vi "CSM Module Template - Tiny.vi"(7 "Name (\"\" to Use UUID)":string="CSM Tiny") -> ()   [LabVIEW 2017]
doc: "Compact code template for creating a CSM module without a user interface. The functionality of this template is identical to the CSM Module Template VI.\n\n\n> [!NOTE] <b>CSM Naming Rules</b>\n>\n> - CSM module name must be unique. Otherwise, CSM enters a `Critical Error` state.\n> - If the input module name is an empty string (\"\"), the system uses a UUID as the module name. Such a module is marked as standalone mode and does not appear in the module list.\n> - Worker Mode Rule: If the input module name ends with `#`, a worker mode node will be instantiated. Multiple worker mode nodes can form a worker mode module.\n> - Chain of Responsibility Mode Rule: If the input module name ends with `$` followed by a number, a chain of responsibility mode node will be instantiated. Multiple chain of responsibility mode nodes can form a chain of responsibility mode module.\n> - System-Level Module Rule: If the input module name starts with `.`, the module is a system-level module. Under default settings, such modules are not listed by the CSM - List Modules VI and are suitable for instantiating modules that run in the background.\n> - Submodule Rule: `.` is also allowed in a module name to separate the module name into multiple parts. CSM does not have strict rules for submodules. The `.` in the module name only marks the logical relationship between different modules. From an execution perspective, they are considered independent modules. The only difference is that you can obtain a list of logical submodules via the CSM - List Submodules VI.\n\n\n-- <b>Controls</b> --\n- <b>Name (\"\" to use UUID)</b>: CSM module name. Refer to <b>CSM Naming Rules</b> for module naming rules."
uses:
  user.lib/_NEVSTOP/Communicable State Machine(CSM)/AdvanceAPI/CSM - Revert Arguments-Safe String.vi
  user.lib/_NEVSTOP/Communicable State Machine(CSM)/AdvanceAPI/CSM - Break Down Multiple States String.vi
  user.lib/_NEVSTOP/Communicable State Machine(CSM)/AdvanceAPI/CSM - Compact Multiple States.vi
  user.lib/_NEVSTOP/Communicable State Machine(CSM)/AdvanceAPI/CSM - Make String Arguments Safe.vi
  user.lib/_NEVSTOP/Communicable State Machine(CSM)/AdvanceAPI/CSM - Keywords.vi
  user.lib/_NEVSTOP/Communicable State Machine(CSM)/_Shared/Trim Single-line Text.vi
  user.lib/_NEVSTOP/Communicable State Machine(CSM)/Communicable State Machine.lvlib
panel:
  in  "Exit":bool
  out "State History":string
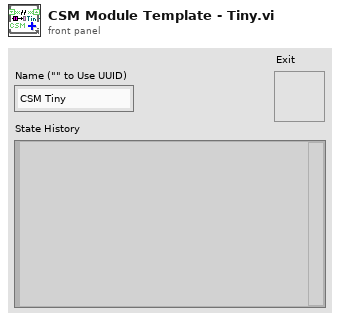
[diagram p1: front panel]
types:
  T1 = enum32{"Invalid", "Standard", "Closed", "Hidden", "Minimized", "Maximized"}
  T2 = enum32{"invalid app kind", "Development System", "Run Time System", "Student Edition", "Embedded LabVIEW", "Evaluation", "Custom"}
  T3 = typedef "Communicable State Machine.lvlib/_CSM_Response Source Message.ctl" = cluster{"‘State":string, "’Arguments":string, "’Error":errorcluster}
  T4 = cluster{"Current VI Reference":refnum<vi>, "Close Panel on Exit?":bool}
  T5 = cluster{"Core":cluster{"Current VI Reference":refnum<vi>, "Close Panel on Exit?":bool}, "Your Boolean data":bool, "Your string data":string}
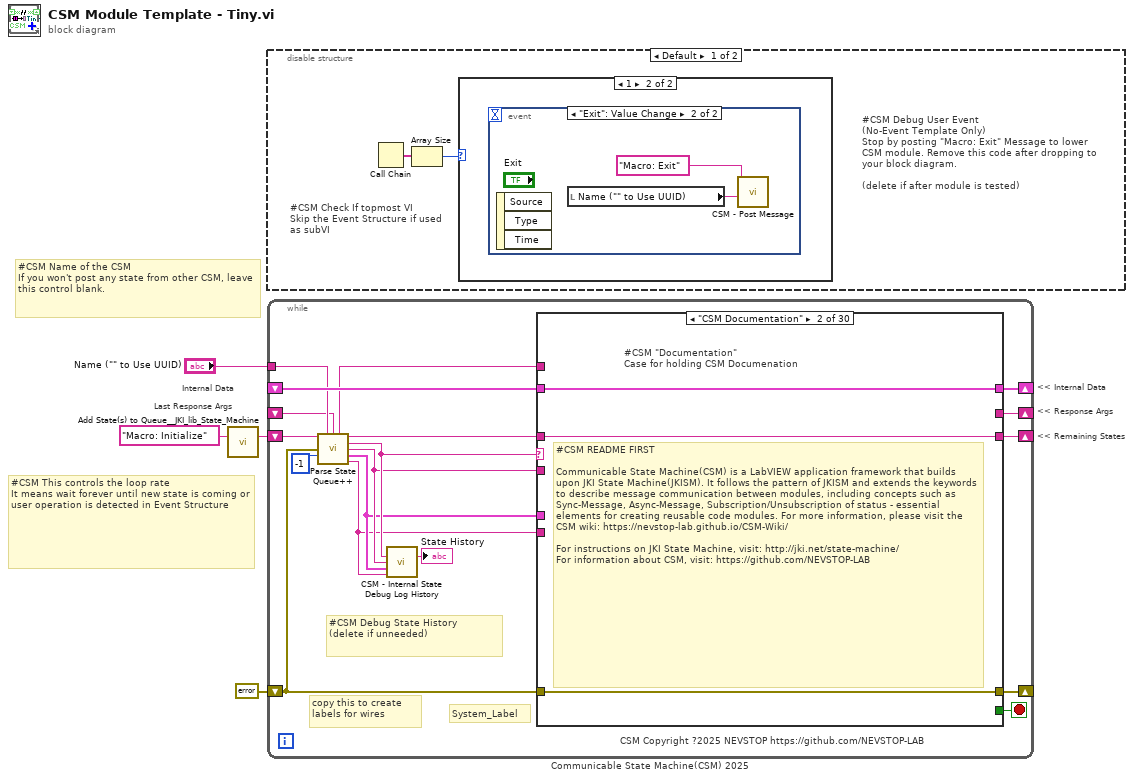
[diagram p0: block diagram]
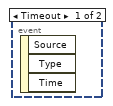
[diagram p3: hidden frame]
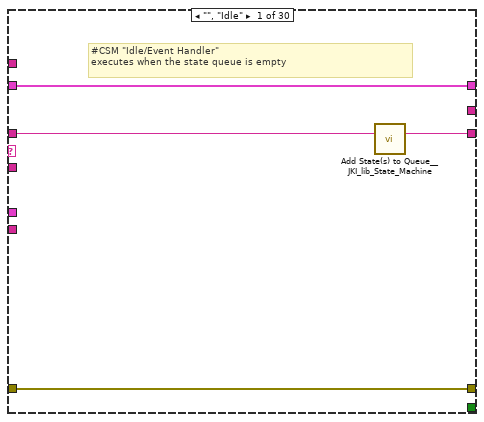
[diagram p5: hidden frame]
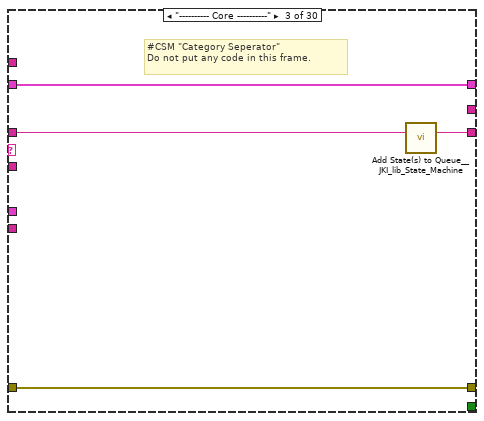
[diagram p6: hidden frame]
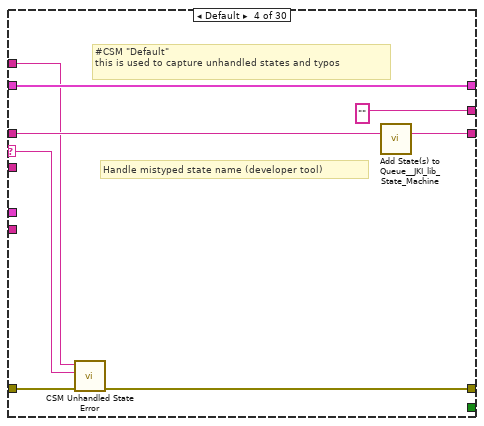
[diagram p7: hidden frame]
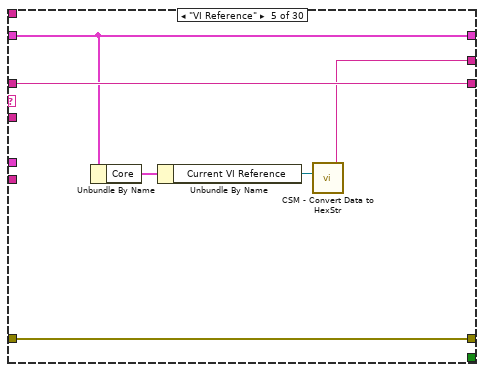
[diagram p8: hidden frame]
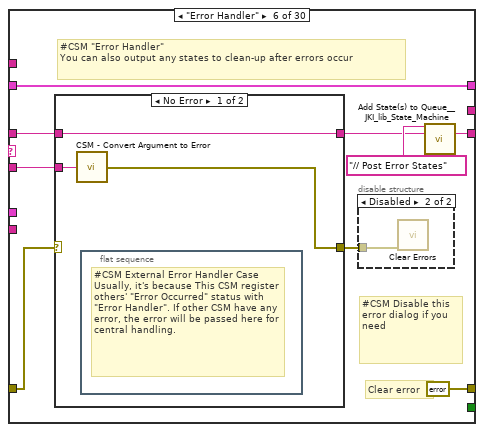
[diagram p9: hidden frame]
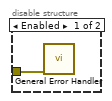
[diagram p10: hidden frame]
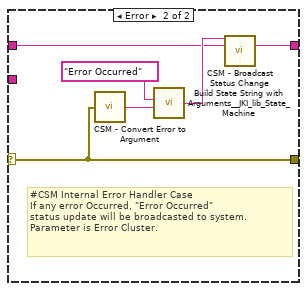
[diagram p11: hidden frame]
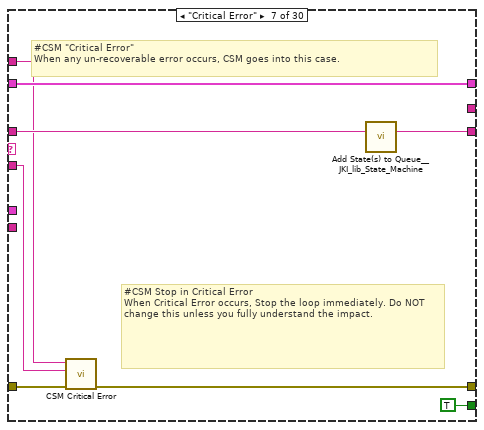
[diagram p12: hidden frame]
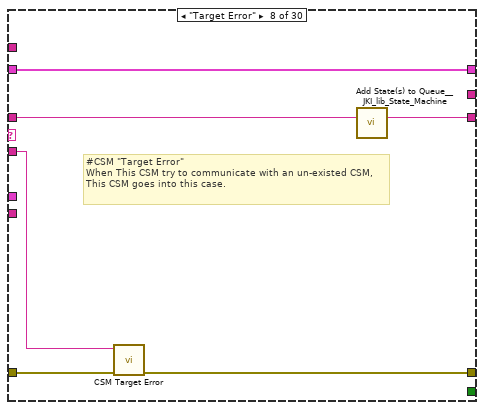
[diagram p13: hidden frame]
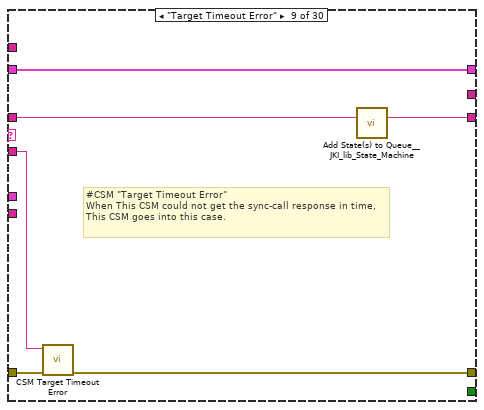
[diagram p14: hidden frame]
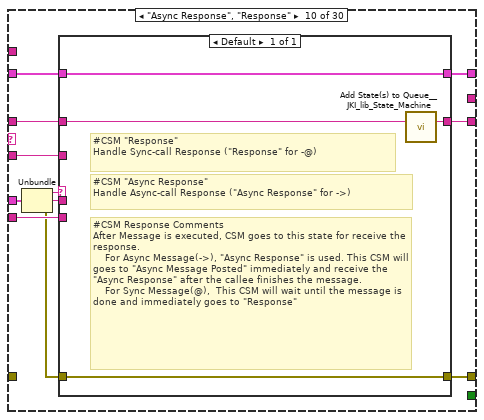
[diagram p15: hidden frame]
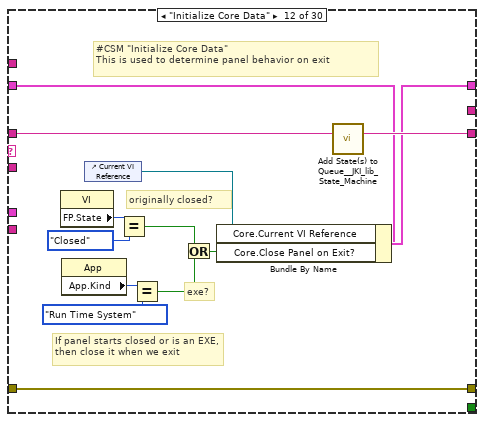
[diagram p17: hidden frame]
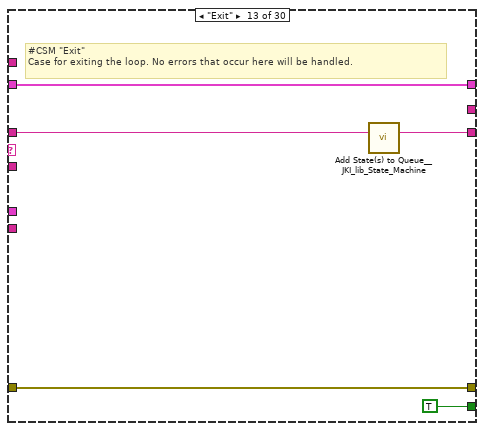
[diagram p18: hidden frame]
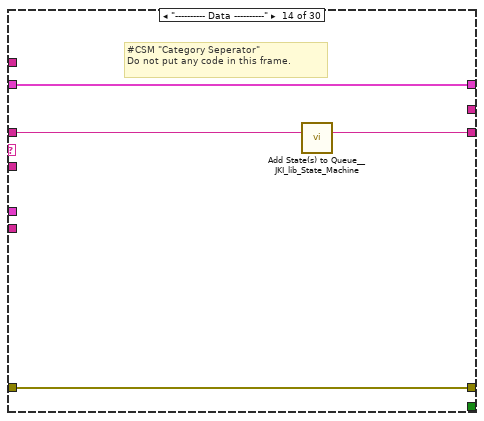
[diagram p19: hidden frame]
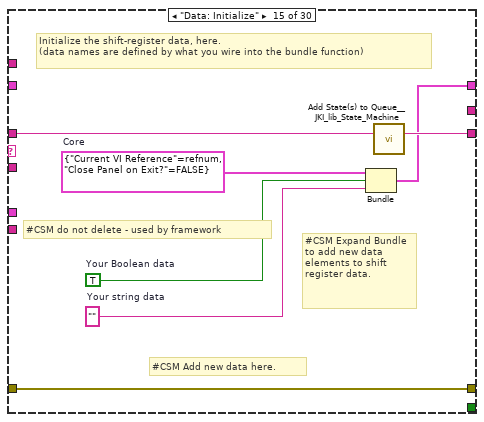
[diagram p20: hidden frame]
diagram:
  # "Last Response Args"
  # "Internal Data"
  # "#CSM Name of the CSM\nIf you won't post any state from other CSM, leave this control blank."
  # "#CSM This controls the loop rate\nIt means wait forever until new state is coming or user operation is detected in Event Structure"
  # "<< Internal Data"
  # "<< Response Args"
  # "<< Remaining States"
  n1 = call <vilib>:"Add State(s) to Queue__JKI_lib_State_Machine.vi"("State(s) in (\"\")"="Macro: Initialize" ("Init State(\"Macro: Initialize\")")) -> ("States Out"=w4:string)  [unwired: 14 in]
  n2 = disable-structure shown="Default" {
    frame condition #0 (active) {
      # "#CSM Check If topmost VI\nSkip the Event Structure if used as subVI"
      # "#CSM Debug User Event\n(No-Event Template Only)\nStop by posting \"Macro: Exit\" Message to lower CSM module. Remove this code after dropping to your block diagram. \n\n(delete if after module is tested)"
      n3 = Call Chain() -> (call chain=w6:string[])
      n4 = Array Size(array=w6) -> (size(s)=w5:i32)
      n5 = case shown="1" w5 {
        frame Default {
        }
        frame 1 {
          n6 = event shown="[1] \"Exit\": Value Change" {
            selector: _ -> [_ _]
            dyn-events: _ -> [_ _]
            timeout: _ -> [_ _]
            event Timeout {
              n7 = event-data() -> ()  [unwired: 1 in, 3 out]
            }
            event "Exit": Value Change {
              n8 = event-data() -> ()  [unwired: 1 in, 3 out]
              n9 = local read "Name (\"\" to Use UUID)"() -> (w8:string)
              n10 = call "CSM - Post Message.vi"("Target Module"=w8, "State"="Macro: Exit" ("States")) -> ()  [unwired: 9 in, 1 out]
            }
          }
        }
      }
    }
    frame condition #1 {
    }
  }
  n11 = while "Communicable State Machine(CSM) 2025" {
    shift-right: [w21] -> _
    shift-left: _ -> [w20]
    shift-right: [w24] -> _
    shift-left: errorcluster {"status"=FALSE, "code"=0, "source"=""} ("error out") -> [w19]
    shift-right: [w23] -> _
    shift-left: w4 -> [w25]
    tunnel: "Name (\"\" to Use UUID)" -> [w17]
    shift-right: [w18] -> _
    shift-left: _ -> [w11]
    stop <- w22 stop-if-true
    # "#CSM Debug State History\n(delete if unneeded)"
    # "copy this to create labels for wires"
    # "System_Label"
    # "CSM Copyright ?2025 NEVSTOP https://github.com/NEVSTOP-LAB"
    n12 = call "Parse State Queue++.vi"("State Queue"=w25, "Name (\"\" to Use UUID)"=w17, "Response Arguments"=w11, "Previous Error"=w19, "Dequeue (1 ms)"=-1 ("Timeout")) -> ("Name Used"=w12:string, "Remaining States"=w26:string, "Current State"=w16:string, "Arguments"=w15:string, "Additional Information"=w14:T3, "Source CSM"=w13:string)  [unwired: 5 in]
    n13 = call "CSM - Internal State Debug Log History.vi"("State"=w16, "Arguments (\"\")"=w15, ">> Response Source Message >>"=w14, "Source (\"\")"=w13) -> ("Debug Log"=→"State History":string)  [unwired: 11 in]
    n14 = case shown="\"CSM Documentation\"" w16 {
      selector: w16 -> [_ _ _ w40 _ _ _ _ _ _ _ _ _ _ _ _ _ _ _ _ _ _ _ _ _ _ _ _ _ _]
      tunnel: w26 -> [w27 w32 w37 w44 w50 w56 w77 w83 w89 w97 w108 w122 w127 w131 w138 w140 w147 w151 w155 w161 w176 w245 w250 w257 w259 w263 w268 w275 w279 w283]
      tunnel: w15 -> [_ _ _ _ _ w55 w73 w82 w87 w96 _ _ _ _ _ _ _ _ _ w156 w170 _ _ _ _ _ w266 _ _ _]
      tunnel: w20 -> [w28 w31 w34 w42 w49 w59 w78 w84 w90 w99 w107 w115 w125 w128 _ w139 w142 w148 w153 w159 w172 w242 w247 w254 w258 w262 w267 w272 w276 w280]
      tunnel: [w29 w33 w35 w38 w51 errorcluster {"status"=FALSE, "code"=0, "source"=""} ("error out") w74 w80 w86 w102 w109 w119 w124 w129 w135 w141 w143 w149 w152 w157 w173 w243 w248 w255 w260 w264 w269 w273 w277 w281] -> w24
      tunnel: w19 -> [w29 w33 w35 w45 w51 w57 w79 w81 w88 _ w109 w119 w124 w129 w135 w141 w144 w149 w152 w158 w174 w243 w248 w255 w260 w264 w269 w273 w277 w281]
      tunnel: [w30 w32 w36 w43 w50 w52 w76 w85 w91 w98 w108 w121 w126 w130 w137 w140 w146 w150 w154 w160 w175 w244 w249 w256 w259 w263 w268 w274 w278 w282] -> w23
      tunnel: [_ _ _ _ _ _ TRUE _ _ _ _ _ TRUE _ _ _ _ _ _ _ _ _ _ _ _ _ _ _ _ _] -> w22
      tunnel: [w28 w31 w34 w42 w49 w59 w78 w84 w90 w100 w107 w120 w125 w128 w136 w139 w142 w148 w153 w159 w172 w242 w247 w254 w258 w262 w267 w272 w276 w280] -> w21
      tunnel: w13 -> [_ _ _ _ _ _ _ _ _ w94 _ _ _ _ _ _ _ _ _ _ _ _ _ _ _ _ _ _ _ _]
      tunnel: w14 -> [_ _ _ _ _ _ _ _ _ w101 _ _ _ _ _ _ _ _ _ _ _ _ _ _ _ _ _ _ _ _]
      tunnel: [_ _ _ "" w46 _ _ _ _ _ _ _ _ _ _ _ _ _ _ _ _ _ _ _ _ "API1 Response" w265 _ _ _] -> w18
      tunnel: w12 -> [_ _ _ w39 _ _ w72 _ _ _ _ _ _ _ _ _ _ _ _ _ _ _ _ _ _ _ _ _ _ _]
      frame "", "Idle" {
        # "#CSM \"Idle/Event Handler\"\nexecutes when the state queue is empty"
        n15 = call <vilib>:"Add State(s) to Queue__JKI_lib_State_Machine.vi"("State(s) in (\"\")"=w27) -> ("States Out"=w30:string)  [unwired: 14 in]
      }
      frame "CSM Documentation" {
        # "#CSM README FIRST\n\nCommunicable State Machine(CSM) is a LabVIEW application framework that builds upon JKI State Machine(JKISM). It follows the pattern of JKISM and extends the keywords to describe message communication between modules, including concepts such as Sync-Message, Async-Message, Subscription/Unsubscription of status - essential elements for creating reusable code modules. For more information, please visit the CSM wiki: https://nevstop-lab.github.io/CSM-Wiki/\n\nFor instructions on JKI State Machine, visit: http://jki.net/state-machine/\nFor information about CSM, visit: https://github.com/NEVSTOP-LAB"
        # "#CSM \"Documentation\"\nCase for holding CSM Documenation"
      }
      frame "---------- Core ----------" {
        # "#CSM \"Category Seperator\"\nDo not put any code in this frame."
        n16 = call <vilib>:"Add State(s) to Queue__JKI_lib_State_Machine.vi"("State(s) in (\"\")"=w37) -> ("States Out"=w36:string)  [unwired: 14 in]
      }
      frame Default {
        # "#CSM \"Default\"\nthis is used to capture unhandled states and typos"
        # "Handle mistyped state name (developer tool)"
        n17 = call "CSM Unhandled State Error.vi"("error in (no error)"=w45, "Undefined State"=w40, "CSM Name"=w39) -> ("error out"=w38:errorcluster)  [unwired: 8 in]
        n18 = call <vilib>:"Add State(s) to Queue__JKI_lib_State_Machine.vi"("State(s) in (\"\")"=w44) -> ("States Out"=w43:string)  [unwired: 14 in]
      }
      frame "VI Reference" {
        n19 = Unbundle By Name(w49) -> ("Core"=w48:T4)
        n20 = Unbundle By Name(w48) -> ("Current VI Reference"=w47:refnum<vi>)
        n21 = call "CSM - Convert Data to HexStr.vi"("Variant"=w47) -> ("HEX String (0-9,A-F)"=w46:string)  [unwired: 8 in]
      }
      frame "Error Handler" {
        # "#CSM Disable this error dialog if you need"
        # "#CSM \"Error Handler\"\nYou can also output any states to clean-up after errors occur"
        # "Clear error"
        n22 = case shown="No Error" w57 {
          selector: w57 -> [_ w66]
          tunnel: [w65 w68] -> w53
          tunnel: w56 -> [w65 w67]
          tunnel: w55 -> [w64 _]
          tunnel: [w63 w66] -> w58
          frame No Error {
            n23 = call "CSM - Convert Argument to Error.vi"("Argument"=w64) -> ("Error"=w63:errorcluster)  [unwired: 4 in]
            n24 = flat-sequence {
              frame #0 {
                # "#CSM External Error Handler Case\nUsually, it's because This CSM register others' \"Error Occurred\" status with \"Error Handler\". If other CSM have any error, the error will be passed here for central handling."
              }
            }
          }
          frame Error {
            # "#CSM Internal Error Handler Case \nIf any error Occurred, \"Error Occurred\" \nstatus update will be broadcasted to system.\nParameter is Error Cluster."
            n25 = call "CSM - Convert Error to Argument.vi"("Error"=w66) -> ("Argument"=w70:string)  [unwired: 4 in]
            n26 = call <vilib>:"Build State String with Arguments__JKI_lib_State_Machine.vi"("Arguments (\"\")"=w70, "State"="Error Occurred" ("Status with Arguments")) -> ("State with Arguments"=w69:string)  [unwired: 4 in]
            n27 = call "CSM - Broadcast Status Change.vi"("Status With Arguments"=w69, "State Queue"=w67) -> ("Remaining States"=w68:string)  [unwired: 13 in]
          }
        }
        n28 = disable-structure shown="Disabled" {
          disable-tunnel: w58 -> [w61 w62]
          frame Enabled {
            n29 = call <vilib>:"General Error Handler.vi"("error in (no error)"=w61) -> ()  [unwired: 10 in, 5 out]
          }
          frame Disabled {
            n30 = call <vilib>:"Clear Errors.vi"("error in (no error)"=w62) -> ()  [unwired: 5 in, 2 out]
          }
        }
        n31 = call <vilib>:"Add State(s) to Queue__JKI_lib_State_Machine.vi"("State(s) in Front (\"\")"="// Post Error States", "State(s) in (\"\")"=w53) -> ("States Out"=w52:string)  [unwired: 13 in]
      }
      frame "Critical Error" {
        # "#CSM Stop in Critical Error\nWhen Critical Error occurs, Stop the loop immediately. Do NOT change this unless you fully understand the impact."
        # "#CSM \"Critical Error\"\nWhen any un-recoverable error occurs, CSM goes into this case."
        n32 = call "CSM Critical Error.vi"("error in (no error)"=w79, "Arugments (As Reason)"=w73, "CSM Name"=w72) -> ("error out"=w74:errorcluster)  [unwired: 8 in]
        n33 = call <vilib>:"Add State(s) to Queue__JKI_lib_State_Machine.vi"("State(s) in (\"\")"=w77) -> ("States Out"=w76:string)  [unwired: 14 in]
      }
      frame "Target Error" {
        # "#CSM \"Target Error\"\nWhen This CSM try to communicate with an un-existed CSM, This CSM goes into this case."
        n34 = call "CSM Target Error.vi"("error in (no error)"=w81, "Arguments (As CSM Name)"=w82) -> ("error out"=w80:errorcluster)  [unwired: 9 in]
        n35 = call <vilib>:"Add State(s) to Queue__JKI_lib_State_Machine.vi"("State(s) in (\"\")"=w83) -> ("States Out"=w85:string)  [unwired: 14 in]
      }
      frame "Target Timeout Error" {
        # "#CSM \"Target Timeout Error\"\nWhen This CSM could not get the sync-call response in time, This CSM goes into this case."
        n36 = call "CSM Target Timeout Error.vi"("error in (no error)"=w88, "Arguments (As CSM Name)"=w87) -> ("error out"=w86:errorcluster)  [unwired: 9 in]
        n37 = call <vilib>:"Add State(s) to Queue__JKI_lib_State_Machine.vi"("State(s) in (\"\")"=w89) -> ("States Out"=w91:string)  [unwired: 14 in]
      }
      frame "Async Response", "Response" {
        n38 = Unbundle(w101) -> ("‘State"=w95:string, "’Arguments"=w93:string, "’Error"=w92:errorcluster)
        n39 = case shown="Default" w95 {
          tunnel: [w106] -> w102
          tunnel: w92 -> [w106]
          tunnel: [w105] -> w100
          tunnel: w99 -> [w105]
          tunnel: [w103] -> w98
          tunnel: w97 -> [w104]
          tunnel: w96 -> [_]
          tunnel: w94 -> [_]
          tunnel: w93 -> [_]
          frame Default {
            # "#CSM Response Comments\nAfter Message is executed, CSM goes to this state for receive the response.\n    For Async Message(->), \"Async Response\" is used. This CSM will goes to \"Async Message Posted\" immediately and receive the \"Async Response\" after the callee finishes the message.\n    For Sync Message(@),  This CSM will wait until the message is done and immediately goes to \"Response\""
            # "#CSM \"Async Response\"\nHandle Async-call Response (\"Async Response\" for ->)"
            # "#CSM \"Response\"\nHandle Sync-call Response (\"Response\" for -@)"
            n40 = call <vilib>:"Add State(s) to Queue__JKI_lib_State_Machine.vi"("State(s) in (\"\")"=w104) -> ("States Out"=w103:string)  [unwired: 14 in]
          }
        }
      }
      frame "Async Message Posted" {
        # "#CSM \"Async Message Posted\"\nAfter Async Message is posted (-> or ->| ), CSM goes to this state for post-action.\nYou can use Argument - State to tell which Async Message is called."
      }
      frame "Initialize Core Data" {
        # "#CSM \"Initialize Core Data\"\nThis is used to determine panel behavior on exit"
        # "originally closed?"
        # "exe?"
        # "If panel starts closed or is an EXE, then close it when we exit"
        n41 = property class="VI"() -> ("FP.State"=w112:T1)  [unwired: 2 in, 2 out]
        n42 = property class="App"() -> ("App.Kind"=w118:T2)  [unwired: 2 in, 2 out]
        n43 = control-ref of="Current VI Reference"() -> (w113:refnum<vi>)
        n44 = Equal?(x=w112, y=T1."Closed" ("Front Panel Window:State")) -> (x = y?=w110:bool)
        n45 = Equal?(x=w118, y=T2."Run Time System" ("Application:Kind")) -> (x = y?=w116:bool)
        n46 = Or(x=w110, y=w116) -> (x .or. y?=w114:bool)
        n47 = Bundle By Name(cluster=w115, "Core.Current VI Reference"=w113, "Core.Close Panel on Exit?"=w114) -> (w120:T5)
        n48 = call <vilib>:"Add State(s) to Queue__JKI_lib_State_Machine.vi"("State(s) in (\"\")"=w122) -> ("States Out"=w121:string)  [unwired: 14 in]
      }
      frame "Exit" {
        # "#CSM \"Exit\"\nCase for exiting the loop. No errors that occur here will be handled."
        n49 = call <vilib>:"Add State(s) to Queue__JKI_lib_State_Machine.vi"("State(s) in (\"\")"=w127) -> ("States Out"=w126:string)  [unwired: 14 in]
      }
      frame "---------- Data ----------" {
        # "#CSM \"Category Seperator\"\nDo not put any code in this frame."
        n50 = call <vilib>:"Add State(s) to Queue__JKI_lib_State_Machine.vi"("State(s) in (\"\")"=w131) -> ("States Out"=w130:string)  [unwired: 14 in]
      }
      frame "Data: Initialize" {
        w132 = T4 {"Current VI Reference"=refnum, "Close Panel on Exit?"=FALSE}  # Core
        w134 = TRUE  # Your Boolean data
        w133 = ""  # Your string data
        # "#CSM do not delete - used by framework"
        # "#CSM Expand Bundle to add new data elements to shift register data."
        # "#CSM Add new data here."
        # "Initialize the shift-register data, here.\n(data names are defined by what you wire into the bundle function)"
        n51 = Bundle("Core"=w132, "Your Boolean data"=w134, "Your string data"=w133) -> (w136:T5)  [unwired: 1 in]
        n52 = call <vilib>:"Add State(s) to Queue__JKI_lib_State_Machine.vi"("State(s) in (\"\")"=w138) -> ("States Out"=w137:string)  [unwired: 14 in]
      }
      frame "Data: Update Indicators" {
      }
      frame "Data: Cleanup" {
        # "Cleanup any data and references, here.\n(this is called automatically, by the Macro: Exit)"
        n53 = Unbundle By Name(w142) -> ("Core.Current VI Reference"=w145:refnum<vi>)
        n54 = Close Reference(reference=w145, error in (no error)=w144) -> (error out=w143:errorcluster)
        n55 = call <vilib>:"Add State(s) to Queue__JKI_lib_State_Machine.vi"("State(s) in (\"\")"=w147) -> ("States Out"=w146:string)  [unwired: 14 in]
      }
      frame "---------- UI ----------" {
        # "#CSM \"Category Seperator\"\nDo not put any code in this frame."
        n56 = call <vilib>:"Add State(s) to Queue__JKI_lib_State_Machine.vi"("State(s) in (\"\")"=w151) -> ("States Out"=w150:string)  [unwired: 14 in]
      }
      frame "UI: Initialize" {
        # "#CSM \"UI: Initialize\"\nInitialize the User Interface, here.\n(this is called automatically, by the Macro: Init)"
        n57 = call <vilib>:"Add State(s) to Queue__JKI_lib_State_Machine.vi"("State(s) in (\"\")"=w155) -> ("States Out"=w154:string)  [unwired: 14 in]
      }
      frame "UI: Cursor Set" {
        # "#CSM \"UI: Cursor Set\"\nSet and Unset Cursor Busy.\n(Usage: \"UI: Cursor Set >> Busy|Idle\")"
        # "Argument"
        n58 = disable-structure shown="TARGET_TYPE!=Windows" {
          disable-tunnel: w158 -> [w164 w169]
          disable-tunnel: [w163 w169] -> w157
          disable-tunnel: w156 -> [w162 _]
          frame condition #0 (active) {
            n59 = case shown="\"Idle\", Default" w162 {
              tunnel: w164 -> [w166 w168]
              tunnel: [w165 w167] -> w163
              frame "Idle", Default {
                n60 = call <vilib>:"Unset Busy.vi"("error in (no error)"=w166) -> ("error out"=w165:errorcluster)  [unwired: 10 in]
              }
              frame "Busy" {
                n61 = call <vilib>:"Set Busy.vi"("error in (no error)"=w168) -> ("error out"=w167:errorcluster)  [unwired: 9 in, 1 out]
              }
            }
          }
          frame condition #1 {
          }
        }
        n62 = call <vilib>:"Add State(s) to Queue__JKI_lib_State_Machine.vi"("State(s) in (\"\")"=w161) -> ("States Out"=w160:string)  [unwired: 14 in]
      }
      frame "UI: Front Panel State" {
        # "#CSM \"UI: Front Panel State\"\nSet Front Panel Open or Closed\n(Usage: \"UI: Front Panel State >> Open|Close\")"
        # "Argument"
        n63 = Unbundle By Name(w172) -> ("Core.Current VI Reference"=w171:refnum<vi>)
        n64 = call <vilib>:"Add State(s) to Queue__JKI_lib_State_Machine.vi"("State(s) in (\"\")"=w176) -> ("States Out"=w175:string)  [unwired: 14 in]
        n65 = case shown="\"Close\", \"Closed\"" w170 {
          tunnel: w174 -> [w182 w197 w208 w221 w234]
          tunnel: [w184 w198 w210 w223 w236] -> w173
          tunnel: w171 -> [w183 w195 w209 w222 w235]
          frame "Open", "Standard", Default {
            w177 = T1."Standard" ("State")
            n66 = property class="VI"(reference=w183, error in=w182) -> (reference out=w180:refnum<vi>, error out=w181:errorcluster, "FP.State"=w179:T1)
            n67 = Not Equal?(x=w179, y=w177) -> (x != y?=w178:bool)
            n68 = case shown="True" w178 {
              tunnel: [w188 w190] -> w184
              tunnel: w181 -> [w187 w190]
              tunnel: w180 -> [w186 _]
              tunnel: w177 -> [w185 _]
              frame True {
                n69 = invoke class="VI" method="FP.Open"(reference=w186, error in=w187, "Activate"=TRUE, "State"=w185) -> (error out=w188:errorcluster)  [unwired: 1 in, 4 out]
              }
              frame False {
              }
            }
          }
          frame "Close", "Closed" {
            n70 = property class="VI"(reference=w195, error in=w197) -> (reference out=w194:refnum<vi>, error out=w196:errorcluster, "FP.State"=w192:T1)
            n71 = Not Equal?(x=w192, y=T1."Closed" ("Front Panel Window:State")) -> (x != y?=w191:bool)
            n72 = case shown="False" w191 {
              tunnel: [w199 w202] -> w198
              tunnel: w196 -> [w199 w201]
              tunnel: w194 -> [_ w200]
              frame False {
              }
              frame True {
                n73 = invoke class="VI" method="FP.Close"(reference=w200, error in=w201) -> (error out=w202:errorcluster)  [unwired: 1 in, 2 out]
              }
            }
          }
          frame "Hidden", "Hide" {
            w203 = T1."Hidden" ("State")
            n74 = property class="VI"(reference=w209, error in=w208) -> (reference out=w206:refnum<vi>, error out=w207:errorcluster, "FP.State"=w205:T1)
            n75 = Not Equal?(x=w205, y=w203) -> (x != y?=w204:bool)
            n76 = case shown="True" w204 {
              tunnel: [w214 w215] -> w210
              tunnel: w207 -> [w213 w215]
              tunnel: w206 -> [w212 _]
              tunnel: w203 -> [w211 _]
              frame True {
                n77 = invoke class="VI" method="FP.Open"(reference=w212, error in=w213, "State"=w211) -> (error out=w214:errorcluster)  [unwired: 2 in, 4 out]
              }
              frame False {
              }
            }
          }
          frame "Minimize", "Minimized" {
            w216 = T1."Minimized" ("State")
            n78 = property class="VI"(reference=w222, error in=w221) -> (reference out=w219:refnum<vi>, error out=w220:errorcluster, "FP.State"=w218:T1)
            n79 = Not Equal?(x=w218, y=w216) -> (x != y?=w217:bool)
            n80 = case shown="True" w217 {
              tunnel: [w227 w228] -> w223
              tunnel: w220 -> [w226 w228]
              tunnel: w219 -> [w225 _]
              tunnel: w216 -> [w224 _]
              frame True {
                n81 = invoke class="VI" method="FP.Open"(reference=w225, error in=w226, "State"=w224) -> (error out=w227:errorcluster)  [unwired: 2 in, 4 out]
              }
              frame False {
              }
            }
          }
          frame "Maximize", "Maximized" {
            w229 = T1."Maximized" ("State")
            n82 = property class="VI"(reference=w235, error in=w234) -> (reference out=w232:refnum<vi>, error out=w233:errorcluster, "FP.State"=w231:T1)
            n83 = Not Equal?(x=w231, y=w229) -> (x != y?=w230:bool)
            n84 = case shown="True" w230 {
              tunnel: [w240 w241] -> w236
              tunnel: w233 -> [w239 w241]
              tunnel: w232 -> [w238 _]
              tunnel: w229 -> [w237 _]
              frame True {
                n85 = invoke class="VI" method="FP.Open"(reference=w238, error in=w239, "State"=w237) -> (error out=w240:errorcluster)  [unwired: 2 in, 4 out]
              }
              frame False {
              }
            }
          }
        }
      }
      frame "---------- Macro ----------" {
        # "#CSM \"Category Seperator\"\nDo not put any code in this frame."
        n86 = call <vilib>:"Add State(s) to Queue__JKI_lib_State_Machine.vi"("State(s) in (\"\")"=w245) -> ("States Out"=w244:string)  [unwired: 14 in]
      }
      frame "Macro: Initialize" {
        # "#CSM \"Macro: Initialize\"\nInitialization Macro (This is called once, when the VI starts)"
        n87 = call <vilib>:"Add State(s) to Queue__JKI_lib_State_Machine.vi"("State(s) in Front (\"\")"="Data: Initialize\nInitialize Core Data\nData: Update Indicators", "State(s) in (\"\")"=w250) -> ("States Out"=w249:string)  [unwired: 13 in]
      }
      frame "Macro: Exit" {
        # "#CSM \"Macro: Exit\"\nExit Macro (This is called once, when the VI exits)"
        n88 = call <vilib>:"Add State(s) to Queue__JKI_lib_State_Machine.vi"("State(s) in Front (\"\")"="//Exit Sub-Modules ", "State(s) at Back (\"\")"="Data: Cleanup\nExit") -> ("States Out"=w252:string)  [unwired: 13 in]
        n89 = call <vilib>:"Add State(s) to Queue__JKI_lib_State_Machine.vi"("State(s) in Front (\"\")"=w252, "State(s) in (\"\")"=w257) -> ("States Out"=w256:string)  [unwired: 13 in]
      }
      frame "---------- API ----------" {
        # "#CSM \"Category Seperator\"\nDo not put any code in this frame."
      }
      frame "API: API1" {
        # "#CSM API Example\nCopy/Rename this case for your own API"
        # "#CSM Response\nConnect this to return the response of your API"
        # "#CSM >> Msg/Rep's CSM >>\nIf you need to tell who triggered this state , use this string. If it's this case itself, this string is \"\"."
        # "#CSM >> Arguments >>\nDeal with the parameter if any"
      }
      frame "API: API2" {
        # "#CSM API Example\nCopy/Rename this case for your own API"
        # "unpack Hex String  to Variant\nif complex parameter is needed."
        n90 = call "CSM - Convert HexStr to Data.vi"("HEX String"=w266) -> ()  [unwired: 7 in, 2 out]
        n91 = disable-structure shown="Disabled" {
          disable-tunnel: [w270 "API2 Response"] -> w265
          frame Disabled {
            # "pack variant to hexstr \nif complex response is needed."
            # "complex Response"
            n92 = call "CSM - Convert Data to HexStr.vi"() -> ("HEX String (0-9,A-F)"=w270:string)  [unwired: 9 in]
          }
          frame Enabled {
          }
        }
      }
      frame "---------- Action ----------" {
        # "#CSM \"Category Seperator\"\nDo not put any code in this frame."
        n93 = call <vilib>:"Add State(s) to Queue__JKI_lib_State_Machine.vi"("State(s) in (\"\")"=w275) -> ("States Out"=w274:string)  [unwired: 14 in]
      }
      frame "Action: action1" {
        # "#CSM \"Internal State\"\nThis category is used for holding internal states"
        n94 = call <vilib>:"Add State(s) to Queue__JKI_lib_State_Machine.vi"("State(s) in (\"\")"=w279) -> ("States Out"=w278:string)  [unwired: 14 in]
      }
      frame "Action: action2" {
        # "#CSM \"Internal State\"\nThis category is used for holding internal states"
        n95 = call <vilib>:"Add State(s) to Queue__JKI_lib_State_Machine.vi"("State(s) in (\"\")"=w283) -> ("States Out"=w282:string)  [unwired: 14 in]
      }
    }
  }
